vi "test Parse System Definition to Get Tx Hardware Channel Info.vi"(8 "error in":errorcluster, 11 "TestCase in":refnum<class "Engine.lvclass">) -> (0 "error out":errorcluster, 3 "TestCase out":refnum<class "Engine.lvclass">)   [LabVIEW 2020, in "Engine.lvclass"]
uses:
  Engine.lvclass
  <vilib>/addons/_JKI Toolkits/VI Tester/TestCase.llb/TestCase.lvclass
  niveristand-custom-device-testing-tools/VeriStandTestUtilities/VeriStandTestUtilities.lvlib
  Scripting/Ballard ARINC 429 Scripting.lvlib
  <vilib>/NI VeriStand/Custom Device API/Custom Device Item Ref.ctl
  <vilib>/NI VeriStand/Custom Device API/Custom Device API.lvlib
  <vilib>/NI VeriStand/Custom Device API/Data Reference.ctl
  Shared/Transfer Type.ctl
  <vilib>/NI VeriStand/Custom Device API/Block Data Reference.ctl
  Encoding and Decoding/Encoding.ctl
  Encoding and Decoding/Encoding and Decoding.lvlib
  Shared/Parameter Definition.ctl
  Shared/RT Parameters.ctl
  Shared/Label.ctl
  Shared/RT Label Settings.ctl
  Shared/RT Hardware Channel Settings.ctl
  C:/Program Files (x86)/National Instruments/LabVIEW 2020/vi.lib/addons/_JKI Toolkits/VI Tester/TestCase.llb/TestCase.lvclass
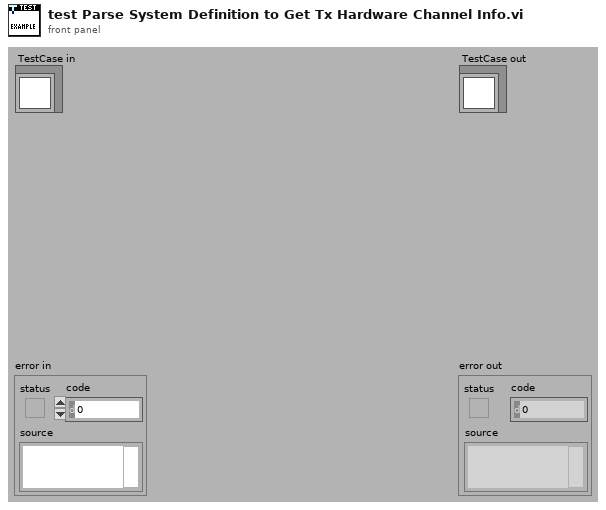
[diagram p1: front panel]
types:
  T1 = typedef "RT Hardware Channel Settings.ctl" = cluster{"channel #":u16, "channel handle":u64, "labels settings for RT":T2[]}
  T2 = typedef "RT Label Settings.ctl" = cluster{"Name":string, "xmlName":string, "label":T3, "transfer period":u32, "SDI_Enabled":bool, "SDI":u8, "parameter driver data":T4, "transfer type":T10, "has timestamp?":bool, "Label Disable/Trigger Channel Reference":T9, "Message Handle":u64, "Initialized?":bool, "Word Initial Raw Value":u32, "Label Timestamp Channel Data Reference":T8, "disabled":bool}
  T3 = typedef "Label.ctl" = u8
  T4 = typedef "RT Parameters.ctl" = cluster{"parameter definitions":T5[], "Rx block data refs":T7[], "Rx values":dbl[], "Tx parameter refs":T9[]}
  T5 = typedef "Parameter Definition.ctl" = cluster{"start index":i32, "size":i32, "encoding":T6, "signed":bool, "scale multiplier":dbl, "scale offset":dbl}
  T6 = typedef "Encoding and Decoding.lvlib/Encoding.ctl" = enum16{"BNR", "BCD", "Discrete"}
  T7 = typedef "Custom Device API.lvlib/Block Data Reference.ctl" = cluster{"Data Reference":T8, "Offset":u64, "Length":u64}
  T8 = typedef "Custom Device API.lvlib/Data Reference.ctl" = i32
  T9 = typedef "Custom Device API.lvlib/Custom Device Item Ref.ctl" = u64
  T10 = typedef "Transfer Type.ctl" = enum16{"Scheduled", "Acyclic", "Block", "Strobe"}
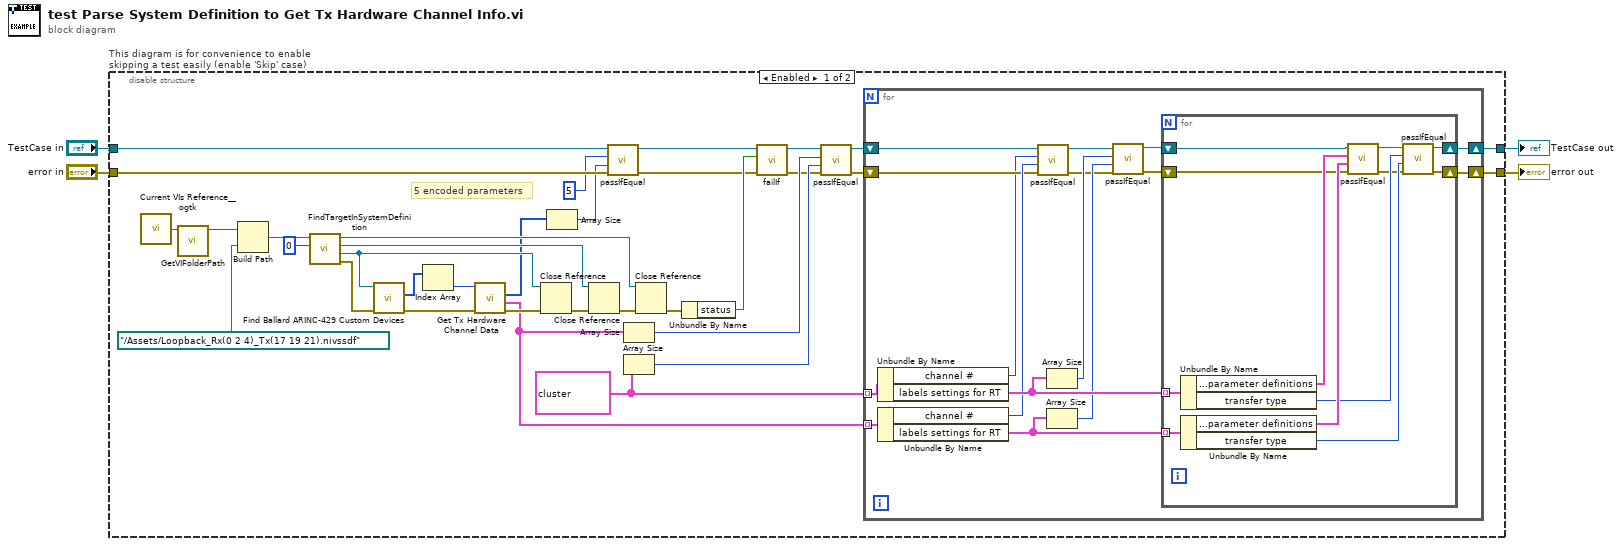
[diagram p0: block diagram]
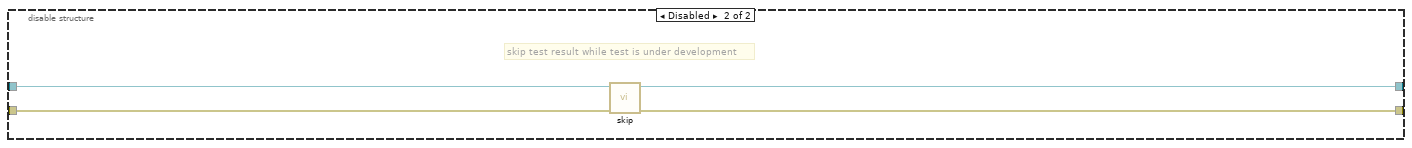
[diagram p2: hidden frame]
diagram:
  n1 = disable-structure "This diagram is for convenience to enable skipping a test easily (enable 'Skip' case)" shown="Enabled" {
    disable-tunnel: "TestCase in" -> [w38 w70]
    disable-tunnel: [w17 w68] -> w1
    disable-tunnel: [w16 w69] -> w3
    disable-tunnel: "error in" -> [w37 w67]
    frame Enabled {
      w20 = T1[] [{"channel #"=17, "channel handle"=0, "labels settings for RT"=[{"Name"="label 134", "xmlName"="134", "label"=134, "transfer period"=0, "SDI_Enabled"=FALSE, "SDI"=0, "parameter driver data"={"parameter definitions"=[{"start index"=18, "size"=10, "encoding"=enum."BNR", "signed"=TRUE, "scale multiplier"=16.0, "scale offset"=0.0}], "Rx block data refs"=[], "Rx values"=[], "Tx parameter refs"=[]}, "transfer type"=enum."Scheduled", "has timestamp?"=FALSE, "Label Disable/Trigger Channel Reference"=18446744073709551615, "Message Handle"=0, "Initialized?"=FALSE, "Word Initial Raw Value"=0, "Label Timestamp Channel Data Reference"=0, "disabled"=FALSE}]}, {"channel #"=19, "channel handle"=0, "labels settings for RT"=[{"Name"="label 135", "xmlName"="135", "label"=135, "transfer period"=0, "SDI_Enabled"=FALSE, "SDI"=0, "parameter driver data"={"parameter definitions"=[{"start index"=10, "size"=19, "encoding"=enum."BCD", "signed"=TRUE, "scale multiplier"=1.0, "scale offset"=0.0}], "Rx block data refs"=[], "Rx values"=[], "Tx parameter refs"=[]}, "transfer type"=enum."Scheduled", "has timestamp?"=FALSE, "Label Disable/Trigger Channel Reference"=18446744073709551615, "Message Handle"=0, "Initialized?"=FALSE, "Word Initial Raw Value"=0, "Label Timestamp Channel Data Reference"=0, "disabled"=FALSE}]}, {"channel #"=21, "channel handle"=0, "labels settings for RT"=[{"Name"="label 136", "xmlName"="136", "label"=136, "transfer period"=0, "SDI_Enabled"=FALSE, "SDI"=0, "parameter driver data"={"parameter definitions"=[{"start index"=13, "size"=16, "encoding"=enum."BNR", "signed"=TRUE, "scale multiplier"=1.0, "scale offset"=0.0}, {"start index"=10, "size"=1, "encoding"=enum."Discrete", "signed"=FALSE, "scale multiplier"=1.0, "scale offset"=0.0}, {"start index"=11, "size"=1, "encoding"=enum."Discrete", "signed"=FALSE, "scale multiplier"=1.0, "scale offset"=0.0}], "Rx block data refs"=[], "Rx values"=[], "Tx parameter refs"=[]}, "transfer type"=enum."Scheduled", "has timestamp?"=FALSE, "Label Disable/Trigger Channel Reference"=18446744073709551615, "Message Handle"=0, "Initialized?"=FALSE, "Word Initial Raw Value"=0, "Label Timestamp Channel Data Reference"=0, "disabled"=FALSE}]}] ("Rx hardware channel data")
      # "5 encoded parameters"
      n2 = call <userlib>:"Current VIs Reference__ogtk.vi"() -> ("Current VI's reference"=w25:refnum<vi>)  [unwired: 5 in]
      n3 = call "GetVIFolderPath.vi"("VI Reference in"=w25) -> ("VI Folder Path out"=w26:path)  [unwired: 9 in, 1 out]
      n4 = Build Path(base path=w26, name or relative path=path "../Assets/Loopback_Rx(0 2 4)_Tx(17 19 21).nivssdf" ("system definition path")) -> (appended path=w24:path)
      n5 = call "FindTargetInSystemDefinition.vi"("target index"=0 ("index"), "system definition path"=w24) -> ("error out"=w30:errorcluster, "Target"=w33:refnum<k24>, "Root"=w32:refnum<k24>, "System Definition"=w31:refnum<k24>)  [unwired: 6 in]
      n6 = call "Find Ballard ARINC-429 Custom Devices.vi"("error in"=w30, "target in"=w33) -> ("error out"=w28:errorcluster, "Ballard ARINC 429 custom devices"=w5:u64[])  [unwired: 7 in, 1 out]
      n7 = Index Array(array=w5) -> (element=w29:u64)  [unwired: 1 in]
      n8 = call "Get Tx Hardware Channel Data.vi"("error in"=w28, "custom device ref in"=w29) -> ("error out"=w27:errorcluster, "Tx hardware channel data"=w21:T1[], "outgoing channels"=w14:T9[])  [unwired: 6 in, 1 out]
      n9 = Close Reference(reference=w33, error in (no error)=w27) -> (error out=w35:errorcluster)
      n10 = Array Size(array=w14) -> (size(s)=w13:i32)
      n11 = Close Reference(reference=w32, error in (no error)=w35) -> (error out=w34:errorcluster)
      n12 = call-dynamic "passIfEqual.vi"("error in (no error)"=w37, "y"=w13, "x"=5 ("size(s)"), "TestCase in"=w38) -> ("error out"=w10:errorcluster, "TestCase out"=w11:refnum<class "Engine.lvclass">)  [unwired: 6 in]
      n13 = Array Size(array=w21) -> (size(s)=w19:i32)
      n14 = Array Size(array=w20) -> (size(s)=w18:i32)
      n15 = Close Reference(reference=w31, error in (no error)=w34) -> (error out=w23:errorcluster)
      n16 = Unbundle By Name(w23) -> ("status"=w22:bool)
      n17 = call-dynamic "failIf.vi"("error in (no error)"=w10, "fail"=w22, "TestCase in"=w11) -> ("error out"=w8:errorcluster, "TestCase out"=w9:refnum<class "Engine.lvclass">)  [unwired: 7 in]
      n18 = call-dynamic "passIfEqual.vi"("error in (no error)"=w8, "y"=w18, "x"=w19, "TestCase in"=w9) -> ("error out"=w6:errorcluster, "TestCase out"=w7:refnum<class "Engine.lvclass">)  [unwired: 6 in]
      n19 = for {
        tunnel: w20 -> [w54] mode=indexing
        tunnel: w21 -> [w53] mode=indexing
        shift-right: [w40] -> w17
        shift-left: w7 -> [w49]
        shift-right: [w41] -> w16
        shift-left: w6 -> [w48]
        n20 = Unbundle By Name(w54) -> ("channel #"=w39:u16, "labels settings for RT"=w52:T2[])
        n21 = Unbundle By Name(w53) -> ("channel #"=w50:u16, "labels settings for RT"=w51:T2[])
        n22 = call-dynamic "passIfEqual.vi"("error in (no error)"=w48, "y"=w50, "x"=w39, "TestCase in"=w49) -> ("error out"=w44:errorcluster, "TestCase out"=w45:refnum<class "Engine.lvclass">)  [unwired: 6 in]
        n23 = Array Size(array=w52) -> (size(s)=w47:i32)
        n24 = Array Size(array=w51) -> (size(s)=w46:i32)
        n25 = call-dynamic "passIfEqual.vi"("error in (no error)"=w44, "y"=w46, "x"=w47, "TestCase in"=w45) -> ("error out"=w42:errorcluster, "TestCase out"=w43:refnum<class "Engine.lvclass">)  [unwired: 6 in]
        n26 = for {
          tunnel: w52 -> [w66] mode=indexing
          tunnel: w51 -> [w65] mode=indexing
          shift-right: [w56] -> w40
          shift-left: w43 -> [w58]
          shift-right: [w55] -> w41
          shift-left: w42 -> [w57]
          n27 = Unbundle By Name(w66) -> ("parameter driver data.parameter definitions"=w64:T5[], "transfer type"=w62:T10)
          n28 = Unbundle By Name(w65) -> ("parameter driver data.parameter definitions"=w63:T5[], "transfer type"=w61:T10)
          n29 = call-dynamic "passIfEqual.vi"("error in (no error)"=w57, "y"=w63, "x"=w64, "TestCase in"=w58) -> ("error out"=w59:errorcluster, "TestCase out"=w60:refnum<class "Engine.lvclass">)  [unwired: 6 in]
          n30 = call-dynamic "passIfEqual.vi"("error in (no error)"=w59, "y"=w61, "x"=w62, "TestCase in"=w60) -> ("error out"=w55:errorcluster, "TestCase out"=w56:refnum<class "Engine.lvclass">)  [unwired: 6 in]
        }
      }
    }
    frame Disabled {
      # "skip test result while test is under development"
      n31 = call <vilib>:"skip.vi"("error in (no error)"=w67, "TestCase in"=w70) -> ("error out"=w69:errorcluster, "TestCase out"=w68:refnum<class "Engine.lvclass">)  [unwired: 8 in]
    }
  }
  "error out" <- w3
  "TestCase out" <- w1
